vi "test_open_close.vi"(8 "error in (no error)":errorcluster) -> (0 "error out":errorcluster)   [LabVIEW 2023, in "Easy.SequenceManager.Test.lvlib"]
uses:
  Easy.SequenceManager.Test.lvlib
  src/SequenceManager/SequenceManager.lvclass
  <vilib>/addons/_JKI Toolkits/Caraya/classes/Assert/Assert Not Error.vi
  <vilib>/addons/_JKI Toolkits/Caraya/classes/Assert/Assert Equal Value_Variant.vi
  <vilib>/addons/_JKI Toolkits/Caraya/classes/Test/Test.lvclass
  <vilib>/addons/_JKI Toolkits/Caraya/classes/Assert/Assert.lvclass
panel:
  in  "SequenceManager in":refnum<class "SequenceManager.lvclass">
  # "Connector Pane"
  # "Locals"
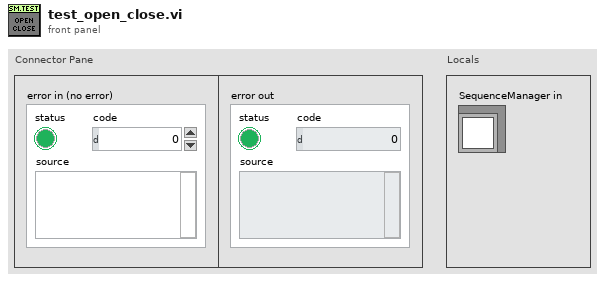
[diagram p1: front panel]
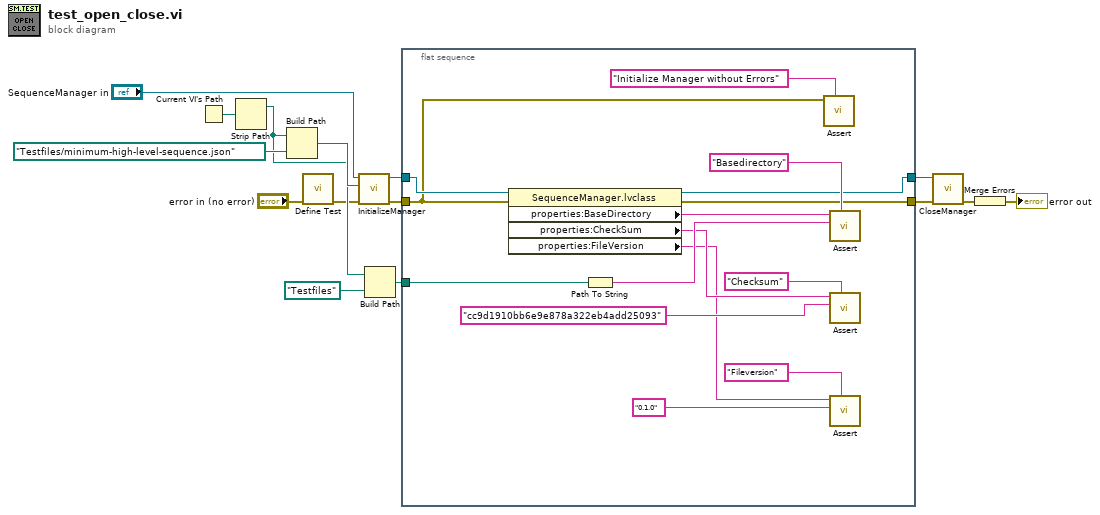
[diagram p0: block diagram]
diagram:
  n1 = Current VI's Path() -> (path=w14:path)
  n2 = Strip Path(path=w14) -> (stripped path=w8:path)  [unwired: 1 out]
  n3 = Build Path(base path=w8, name or relative path=path "Testfiles/minimum-high-level-sequence.json") -> (appended path=w9:path)
  n4 = call <vilib>:"Define Test.vi"("error in (no error)"="error in (no error)") -> ("error out"=w5:errorcluster)  [unwired: 9 in, 1 out]
  n5 = call-dynamic "InitializeManager.vi"("error in (no error)"=w5, "Path to JSON sequence file"=w9, "SequenceManager in"="SequenceManager in") -> ("error out"=w4:errorcluster, "SequenceManager out"=w10:refnum<class "SequenceManager.lvclass">)  [unwired: 7 in]
  n6 = Build Path(base path=w8, name or relative path=path "Testfiles") -> (appended path=w6:path)
  n7 = flat-sequence {
    tunnel: w10 -> [w30]
    tunnel: w6 -> [w28]
    tunnel: w4 -> [w19]
    tunnel: [w18] -> w3
    tunnel: [w17] -> w2
    frame #0 {
      n8 = property class="SequenceManager.lvclass"(reference=w30, error in=w19) -> (reference out=w17:refnum<class "SequenceManager.lvclass">, error out=w18:errorcluster, "properties:BaseDirectory"=w29:string, "properties:CheckSum"=w26:string, "properties:FileVersion"=w21:string)
      n9 = Path To String(path=w28) -> (string=w27:string)
      n10 = call-poly <vilib>:"Assert.vi"("Label"="Initialize Manager without Errors" ("Label (VI Title)"), "Not Error?"=w19) -> ()  [unwired: 8 in, 2 out]
      n11 = call-poly <vilib>:"Assert.vi"("Label"="Basedirectory", "Y"=w27, "X"=w29) -> ()  [unwired: 7 in, 2 out]
      n12 = call-poly <vilib>:"Assert.vi"("Label"="Checksum", "Y"="cc9d1910bb6e9e878a322eb4add25093" ("CheckSum"), "X"=w26) -> ()  [unwired: 7 in, 2 out]
      n13 = call-poly <vilib>:"Assert.vi"("Label"="Fileversion", "Y"="0.1.0" ("FileVersion"), "X"=w21) -> ()  [unwired: 7 in, 2 out]
    }
  }
  n14 = call-dynamic "CloseManager.vi"("error in (no error)"=w3, "SequenceManager in"=w2) -> ("error out"=w1:errorcluster)  [unwired: 8 in, 1 out]
  n15 = Merge Errors(w1) -> (→"error out":errorcluster)
